vi "LPF2Comm.vi"() -> ()   [LabVIEW 2016]
uses:
  VIs/uPythonX/uPythonX.xctl
panel:
  out "Console":string
  in  "stop":bool
  in  "LPF2Class":T1(xcontrol)={"VISA Refnum in"="ASRL23::INSTR", "Python Code"="import machine, utime, gc\n\ndef send_value(data):\n     value = (data & 0xFF)\n     payload = bytes([0xC0, value, 0xFF ^ 0xC0 ^ value])\n     uart.write(payload)\n     print(payload)\n\ntx = machine.Pin('Y9', machine.Pin.OUT)\nrx = machine.Pin('Y10', machine.Pin.IN)\ntx.value(0)\nutime.sleep_ms(500)\ntx.value(1)\n\nuart = machine.UART(3)\nuart.init(baudrate=2400, bits=8, parity=None, stop=1)\n\nuart.write(b'\\x00')\nuart.write(b'\\x40\\x23\\x9C')  #CMD_TYPE (x40)  Type   checksum\nuart.write(b'\\x49\\x02\\x01\\xB5')  #CMD_MODE (x49)  # Modes  # Views   checksum\nuart.write(b'\\x52\\x00\\xC2\\x01\\x00\\x6E')  #CMD_SPEED (x52)  baud (LSB first)   checksum\nuart.write(b'\\x5F\\x00\\x00\\x00\\x02\\x00\\x00\\x00\\x02\\xA0')  #CMD_VERSION (x5F)  Hardware_V  Software_V   checksum\nuart.write(b'\\x9A\\x00\\x4C\\x50\\x46\\x32\\x2D\\x43\\x41\\x4C\\x6E')  #CMD_INFO|bytes|mode  0 name 0   checksum\nuart.write(b'\\x9A\\x01\\x00\\x00\\x00\\x00\\x00\\xC0\\x7F\\x44\\x9F')  #CMD_INFO|3|mode  1 (raw) raw_min  raw_max   checksum\nuart.write(b'\\x9A\\x02\\x00\\x00\\x00\\x00\\x00\\x00\\xC8\\x42\\xED')  #CMD_INFO|3|mode  2 (pct) pct_min  pct_max   checksum\nuart.write(b'\\x9A\\x03\\x00\\x00\\x00\\x00\\x00\\xC0\\x7F\\x44\\x9D')  #CMD_INFO|3|mode  3 (SI) si_min  si_max   checksum\nuart.write(b'\\x92\\x04\\x52\\x41\\x57\\x00\\x2D')  #CMD_INFO|size|mode  0,4,symbol   checksum\nuart.write(b'\\x8A\\x05\\x10\\x00\\x60')  #CMD_INFO|1|mode  5 (FM) Function Map-In   -out   checksum\nuart.write(b'\\x92\\x80\\x03\\x01\\x03\\x00\\xEC')  #CMD_INFO|2|mode  x80 sample_size   Data_type   Figures   Decimals   checksum\nutime.sleep_ms(5)\nprint(uart.read(uart.any()))\nuart.write(b'\\xA1\\x00\\x4C\\x50\\x46\\x32\\x2D\\x43\\x4F\\x55\\x4E\\x54\\x00\\x00\\x00\\x00\\x00\\x00\\x58')  #CMD_INFO|bytes|mode  0 name 0   checksum\nuart.write(b'\\x99\\x01\\x00\\x00\\x00\\x00\\x00\\x00\\xC8\\x42\\xED')  #CMD_INFO|3|mode  1 (raw) raw_min  raw_max   checksum\nuart.write(b'\\x99\\x02\\x00\\x00\\x00\\x00\\x00\\x00\\xC8\\x42\\xEE')  #CMD_INFO|3|mode  2 (pct) pct_min  pct_max   checksum\nuart.write(b'\\x99\\x03\\x00\\x00\\x00\\x00\\x00\\x00\\xC8\\x42\\xEF')  #CMD_INFO|3|mode  3 (SI) si_min  si_max   checksum\nuart.write(b'\\x91\\x04\\x43\\x4E\\x54\\x00\\x33')  #CMD_INFO|size|mode  0,4,symbol   checksum\nuart.write(b'\\x89\\x05\\x10\\x00\\x63')  #CMD_INFO|1|mode  5 (FM) Function Map-In   -out   checksum\nuart.write(b'\\x91\\x80\\x01\\x02\\x04\\x00\\xE9')  #CMD_INFO|2|mode  x80 sample_size   Data_type   Figures   Decimals   checksum\nutime.sleep_ms(5)\nprint(uart.read(uart.any()))\nuart.write(b'\\xA0\\x00\\x4C\\x50\\x46\\x32\\x2D\\x44\\x45\\x54\\x45\\x43\\x54\\x00\\x00\\x00\\x00\\x00\\x1D')  #CMD_INFO|bytes|mode  0 name 0   checksum\nuart.write(b'\\x98\\x01\\x00\\x00\\x00\\x00\\x00\\x00\\x20\\x41\\x07')  #CMD_INFO|3|mode  1 (raw) raw_min  raw_max   checksum\nuart.write(b'\\x98\\x02\\x00\\x00\\x00\\x00\\x00\\x00\\xC8\\x42\\xEF')  #CMD_INFO|3|mode  2 (pct) pct_min  pct_max   checksum\nuart.write(b'\\x98\\x03\\x00\\x00\\x00\\x00\\x00\\x00\\x20\\x41\\x05')  #CMD_INFO|3|mode  3 (SI) si_min  si_max   checksum\nuart.write(b'\\x80\\x04\\x00\\x7B')  #CMD_INFO|size|mode  0,4,symbol   checksum\nuart.write(b'\\x88\\x05\\x10\\x00\\x62')  #CMD_INFO|1|mode  5 (FM) Function Map-In   -out   checksum\nuart.write(b'\\x90\\x80\\x01\\x00\\x03\\x00\\xED')  #CMD_INFO|2|mode  x80 sample_size   Data_type   Figures   Decimals   checksum\nutime.sleep_ms(5)\nprint(uart.read(uart.any()))\nuart.write(b'\\x04')  #ACK\n\n# wait for ACK\nstarttime = utime.time()\ncurrenttime = starttime\n\n# Check for ACK reply\n\nwhile (currenttime-starttime) < 2000:\n     utime.sleep_ms(5)\n     data = uart.read(uart.any())\n     if data.find(b'\\x04') >= 0:\n          print('Success')\n          currenttime = starttime+3000   # stop the loop\n     else:\n          currenttime = utime.time()\n\n# Reset Serial to High Speed\n\n# pull pin low\nuart.deinit()\ntx = machine.Pin('Y9', machine.Pin.OUT)\ntx.value(0)\nutime.sleep_ms(10)\n\n#change baudrate\n\nuart.init(baudrate=115200, bits=8, parity=None, stop=1)\n\n# loop from -10 to 10\ni=-10\n\nwhile True:\n     gc.collect()\n     send_value(i)\n     print(i)\n     i += 1\n     if i > 10: i=-10\n     utime.sleep_ms(200)\n"}
  in  "Numeric":u8=80 format="%.0x"
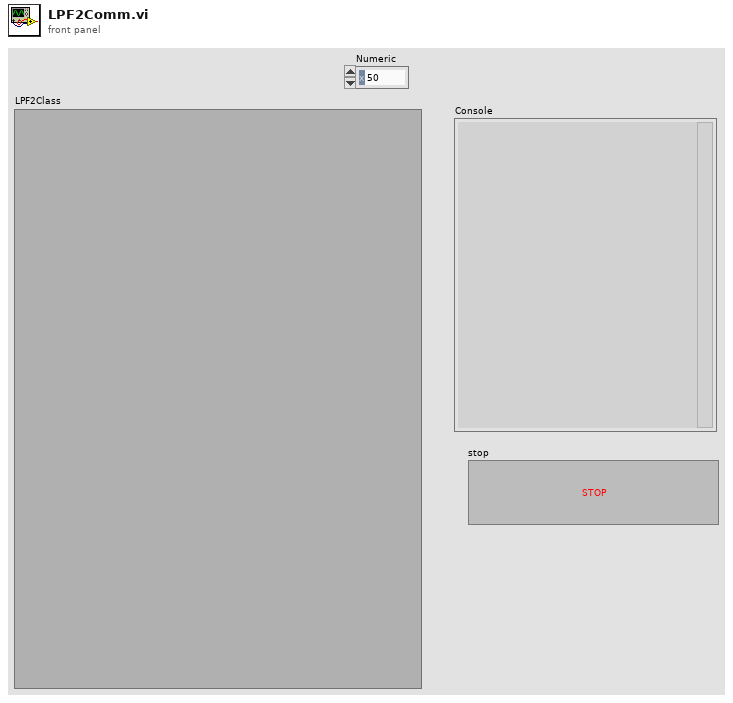
[diagram p1: front panel]
types:
  T1 = cluster{"VISA Refnum in":refnum<visa-resource-name>, "Python Code":string}
  T2 = cluster{"Name":string, "Format":cluster{"# Datasets":u8, "Data Type":u8, "Figures":u8, "Decimals":u8}, "Raw":cluster{"Min":dbl, "Max":dbl}, "Pct":cluster{"Min":dbl, "Max":dbl}, "SI":cluster{"Min":dbl, "Max":dbl}, "Symbol":string, "Funct Map":cluster{"In":u8, "Out":u8}, "view?":bool}[]
  T3 = cluster{"# Datasets":u8, "Data Type":u8, "Figures":u8, "Decimals":u8}
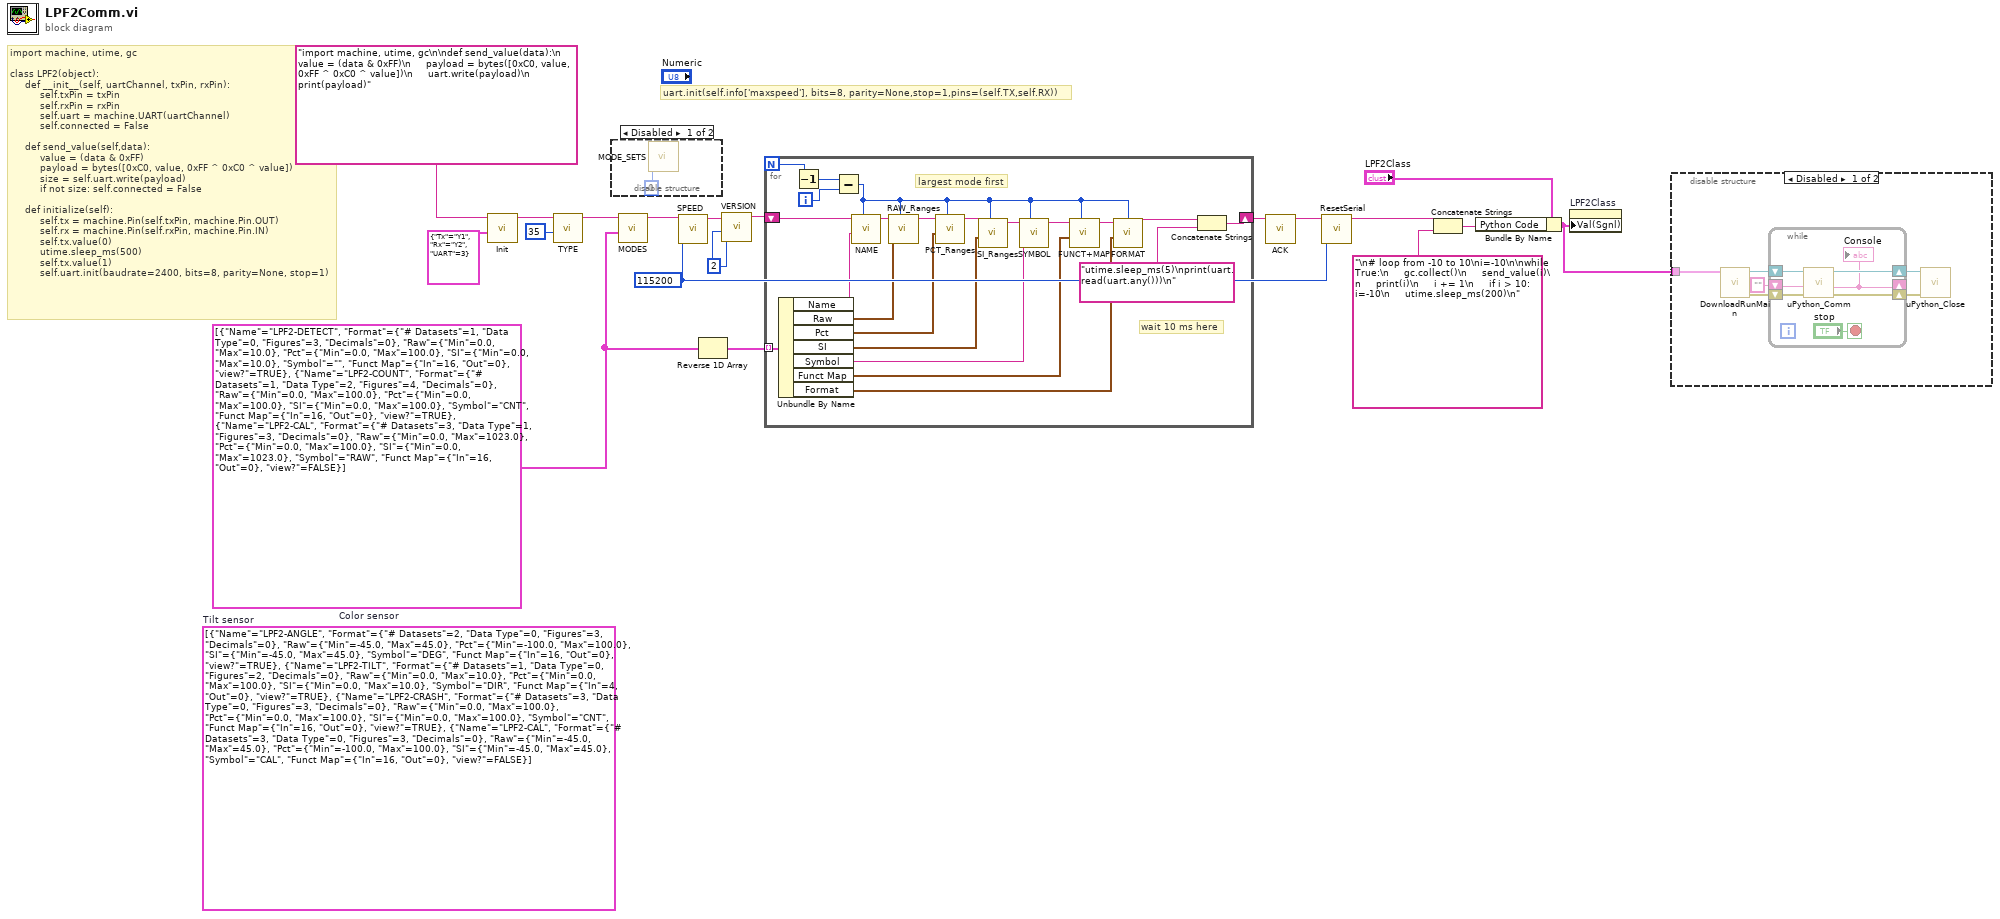
[diagram p0: block diagram]
diagram:
  (unwired) T2 [{"Name"="LPF2-ANGLE", "Format"={"# Datasets"=2, "Data Type"=0, "Figures"=3, "Decimals"=0}, "Raw"={"Min"=-45.0, "Max"=45.0}, "Pct"={"Min"=-100.0, "Max"=100.0}, "SI"={"Min"=-45.0, "Max"=45.0}, "Symbol"="DEG", "Funct Map"={"In"=16, "Out"=0}, "view?"=TRUE}, {"Name"="LPF2-TILT", "Format"={"# Datasets"=1, "Data Type"=0, "Figures"=2, "Decimals"=0}, "Raw"={"Min"=0.0, "Max"=10.0}, "Pct"={"Min"=0.0, "Max"=100.0}, "SI"={"Min"=0.0, "Max"=10.0}, "Symbol"="DIR", "Funct Map"={"In"=4, "Out"=0}, "view?"=TRUE}, {"Name"="LPF2-CRASH", "Format"={"# Datasets"=3, "Data Type"=0, "Figures"=3, "Decimals"=0}, "Raw"={"Min"=0.0, "Max"=100.0}, "Pct"={"Min"=0.0, "Max"=100.0}, "SI"={"Min"=0.0, "Max"=100.0}, "Symbol"="CNT", "Funct Map"={"In"=16, "Out"=0}, "view?"=TRUE}, {"Name"="LPF2-CAL", "Format"={"# Datasets"=3, "Data Type"=0, "Figures"=3, "Decimals"=0}, "Raw"={"Min"=-45.0, "Max"=45.0}, "Pct"={"Min"=-100.0, "Max"=100.0}, "SI"={"Min"=-45.0, "Max"=45.0}, "Symbol"="CAL", "Funct Map"={"In"=16, "Out"=0}, "view?"=FALSE}]  # Tilt sensor
  w9 = T2 [{"Name"="LPF2-DETECT", "Format"={"# Datasets"=1, "Data Type"=0, "Figures"=3, "Decimals"=0}, "Raw"={"Min"=0.0, "Max"=10.0}, "Pct"={"Min"=0.0, "Max"=100.0}, "SI"={"Min"=0.0, "Max"=10.0}, "Symbol"="", "Funct Map"={"In"=16, "Out"=0}, "view?"=TRUE}, {"Name"="LPF2-COUNT", "Format"={"# Datasets"=1, "Data Type"=2, "Figures"=4, "Decimals"=0}, "Raw"={"Min"=0.0, "Max"=100.0}, "Pct"={"Min"=0.0, "Max"=100.0}, "SI"={"Min"=0.0, "Max"=100.0}, "Symbol"="CNT", "Funct Map"={"In"=16, "Out"=0}, "view?"=TRUE}, {"Name"="LPF2-CAL", "Format"={"# Datasets"=3, "Data Type"=1, "Figures"=3, "Decimals"=0}, "Raw"={"Min"=0.0, "Max"=1023.0}, "Pct"={"Min"=0.0, "Max"=100.0}, "SI"={"Min"=0.0, "Max"=1023.0}, "Symbol"="RAW", "Funct Map"={"In"=16, "Out"=0}, "view?"=FALSE}]  # Color sensor
  w13 = u32 115200 ("Baud")
  w14 = u16 2 ("Hardware Version")
  # "import machine, utime, gc\n\nclass LPF2(object):\n     def __init__(self, uartChannel, txPin, rxPin):\n          self.txPin = txPin\n          self.rxPin = rxPin\n          self.uart = machine.UART(uartChannel)\n          self.connected = False\n\n     def send_value(self,data):\n          value = (data & 0xFF)\n          payload = bytes([0xC0, value, 0xFF ^ 0xC0 ^ value])\n          size = self.uart.write(payload)\n          if not size: self.connected = False\n\n     def initialize(self):\n          self.tx = machine.Pin(self.txPin, machine.Pin.OUT)\n          self.rx = machine.Pin(self.rxPin, machine.Pin.IN)\n          self.tx.value(0)\n          utime.sleep_ms(500)\n          self.tx.value(1)\n          self.uart.init(baudrate=2400, bits=8, parity=None, stop=1)"
  # "uart.init(self.info['maxspeed'], bits=8, parity=None,stop=1,pins=(self.TX,self.RX))"
  n1 = call "Init.vi"("Pins"=cluster{"Tx":string, "Rx":string, "UART":i8} {"Tx"="Y1", "Rx"="Y2", "UART"=3}, "Python in"="import machine, utime, gc\n\ndef send_value(data):\n     value = (data & 0xFF)\n     payload = bytes([0xC0, value, 0xFF ^ 0xC0 ^ value])\n     uart.write(payload)\n     print(payload)") -> ("Python out"=w2:string)  [unwired: 9 in]
  n2 = call "TYPE.vi"("Type"=u8 35, "Python in"=w2) -> ("Python out"=w17:string)  [unwired: 9 in]
  n3 = disable-structure shown="Disabled" {
    frame Disabled {
      n4 = call "MODE_SETS.vi"("Mode"=u8 0) -> ()  [unwired: 10 in, 1 out]
    }
    frame Enabled {
    }
  }
  n5 = call "MODES.vi"("Definitions"=w9, "Python in"=w17) -> ("Python out"=w10:string)  [unwired: 9 in]
  n6 = call "SPEED.vi"("Baud"=w13, "Python in"=w10) -> ("Python out"=w16:string)  [unwired: 9 in]
  n7 = Reverse 1D Array(array=w9) -> (reversed array=w11:T2)
  n8 = call "VERSION.vi"("Software Version"=w14, "Hardware Version"=w14, "Python in"=w16) -> ("Python out"=w15:string)  [unwired: 8 in]
  n9 = for {
    N -> [w37]
    shift-right: [w21] -> w18
    shift-left: w15 -> [w42]
    tunnel: w11 -> [w39] mode=indexing
    i -> [w41]
    # "largest mode first"
    # "wait 10 ms here"
    n10 = Unbundle By Name(w39) -> ("Name"=w38:string, "Raw"=w36:cluster{"Min":dbl, "Max":dbl}, "Pct"=w27:cluster{"Min":dbl, "Max":dbl}, "SI"=w23:cluster{"Min":dbl, "Max":dbl}, "Symbol"=w29:string, "Funct Map"=w33:cluster{"In":u8, "Out":u8}, "Format"=w34:T3)
    n11 = Decrement(x=w37) -> (x-1=w40:i32)
    n12 = Subtract(x=w40, y=w41) -> (x-y=w24:i32)
    n13 = call "NAME.vi"("mode"=w24, "Name"=w38, "Python in"=w42) -> ("Python out"=w35:string)  [unwired: 8 in]
    n14 = call "RAW_Ranges.vi"("mode"=w24, "Raw"=w36, "Python in"=w35) -> ("Python out"=w28:string)  [unwired: 8 in]
    n15 = call "PCT_Ranges.vi"("mode"=w24, "Raw"=w27, "Python in"=w28) -> ("Python out"=w25:string)  [unwired: 8 in]
    n16 = call "SI_Ranges.vi"("mode"=w24, "Raw"=w23, "Python in"=w25) -> ("Python out"=w26:string)  [unwired: 8 in]
    n17 = call "SYMBOL.vi"("mode"=w24, "Name"=w29, "Python in"=w26) -> ("Python out"=w31:string)  [unwired: 8 in]
    n18 = call "FUNCT+MAP.vi"("mode"=w24, "Funct Map"=w33, "Python in"=w31) -> ("Python out"=w32:string)  [unwired: 8 in]
    n19 = call "FORMAT.vi"("mode"=w24, "Info"=w34, "Python in"=w32) -> ("Python out"=w22:string)  [unwired: 8 in]
    n20 = Concatenate Strings(w22, "utime.sleep_ms(5)\nprint(uart.read(uart.any()))\n" ("Python in")) -> (w21:string)
  }
  n21 = call "ACK.vi"("Python in"=w18) -> ("Python out"=w5:string)  [unwired: 10 in]
  n22 = call "ResetSerial.vi"("Baud"=w13, "Python in"=w5) -> ("Python out"=w8:string)  [unwired: 9 in]
  n23 = Concatenate Strings(w8, "\n# loop from -10 to 10\ni=-10\n\nwhile True:\n     gc.collect()\n     send_value(i)\n     print(i)\n     i += 1\n     if i > 10: i=-10\n     utime.sleep_ms(200)\n" ("Python in")) -> (w6:string)
  n24 = Bundle By Name(cluster="LPF2Class", "Python Code"=w6) -> (w4:T1)
  n25 = property on="LPF2Class" class="uPythonX (strict)"("Val(Sgnl)"=w4) -> ()  [unwired: 2 in, 2 out]
  n26 = disable-structure shown="Disabled" {
    disable-tunnel: w4 -> [w48 _]
    frame Disabled {
      n27 = call "DownloadRunMain.vi"("Data In"=w48) -> ("error out"=w47:errorcluster, "VISA Refnum out"=w46:refnum<visa-resource-name>)  [unwired: 8 in, 1 out]
      n28 = while {
        shift-right: [w53] -> w45
        shift-left: w47 -> [w55]
        shift-right: [w52] -> w44
        shift-left: w46 -> [w54]
        shift-right: [w49] -> _
        shift-left: "" ("Console Out") -> [w50]
        stop <- "stop" stop-if-true
        n29 = call "uPython_Comm.vi"("error in (no error)"=w55, "Console In"=w50, "VISA Refnum in"=w54) -> ("error out"=w53:errorcluster, "Console Out"=w49:string, "VISA out"=w52:refnum<visa-resource-name>)  [unwired: 4 in, 2 out]
        "Console" <- w49
      }
      n30 = call "uPython_Close.vi"("error in"=w45, "VISA  in"=w44) -> ()  [unwired: 8 in, 2 out]
    }
    frame Enabled {
    }
  }
